vi "BombaPresion.vi"() -> ()   [LabVIEW 2010]
uses:
  <vilib>/Platform/TimedLoop/XDataNode/XDataNode.xnode
  <vilib>/Platform/TimedLoop/XDataNode/timing_clust.ctl
  <vilib>/Platform/TimedLoop/XDataNode/nitl_modes.ctl
  <vilib>/Platform/TimedLoop/XDataNode/wakeup.ctl
  <vilib>/Instr/_visa.llb/VISA Configure Serial Port (Instr).vi
  <vilib>/Platform/TimedLoop/XDataNode/XDNodeRunTimeDep.lvlib
panel:
  out "x*y":dbl
  out "Boolean 2":bool
  out "Boolean":bool
  out "var t 2":i32
  out "nivel presion KPa":dbl(slide) scale=35.0..115.0
  out "presion":dynamicdata(graph)
  in  "presion":dbl(slide) caption="set presion KPa" scale=35.0..115.0
  in  "Period                :":i64=1000
  in  "Flow control    :":u16(ring) items=["None"=0, "XON/XOFF"=1, "RTS/CTS"=2, "DTR/DSR"=4]
  in  "Stop bits         :":u16(ring)=10 items=["1.0"=10, "1.5"=15, "2.0"=20]
  in  "Paridad            :":u16(ring) items=["None", "Odd", "Even", "Mark", "Space"]
  in  "Data bits          :":u16=8 min=5 max=8 step=1
  in  "VISA resource : name:":refnum<visa-resource-name>="COM1"
  in  "Baud rate         :":u32=9600
  in  "stop":bool
  out "Read buffer":string
  # "Sistema Riego"
  # "Configuracion Serial"
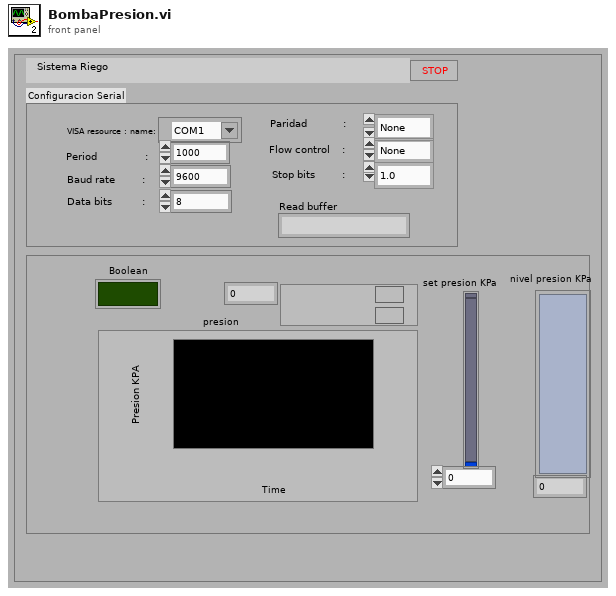
[diagram p1: front panel]
types:
  T1 = typedef "XDNodeRunTimeDep.lvlib/timing_clust.ctl" = cluster{"Expected End [f-1]":u64, "Actual End [f-1]":u64, "Finished Late? [f-1]":bool, "Expected End [i-1]":u64, "Actual End [i-1]":u64, "Finished Late? [i-1]":bool, "Expected Start [i]":u64, "Actual Start [i]":u64, "Expected Start [f]":u64, "Actual Start [f]":u64, "Source Name":string, "Structure Name":string, "Period":i64, "Deadline":i64, "Offset":i64, "Start":i64, "Priority":i32, "Timeout":i32, "Mode":T2, "Wakeup Reason":T3, "Error":errorcluster, "Source Type":string, "Secondary Source Type":string, "Global End Time":u64, "Global Start Time":u64, "Frame Duration":u64, "Iteration Duration":u64, "Assigned CPU":i32, "I/O Scan Engine Mode":u32}
  T2 = typedef "XDNodeRunTimeDep.lvlib/nitl_modes.ctl" = enum32{"No Change", "Process missed periods, maintain original phase", "Discard missed periods, maintain original phase", "Process missed periods, ignore original phase", "Discard missed periods, ignore original phase"}
  T3 = typedef "XDNodeRunTimeDep.lvlib/wakeup.ctl" = enum32{"Normal", "Aborted", "Asynchronous wakeup", "Timing source error", "Timed loop error", "Timeout"}
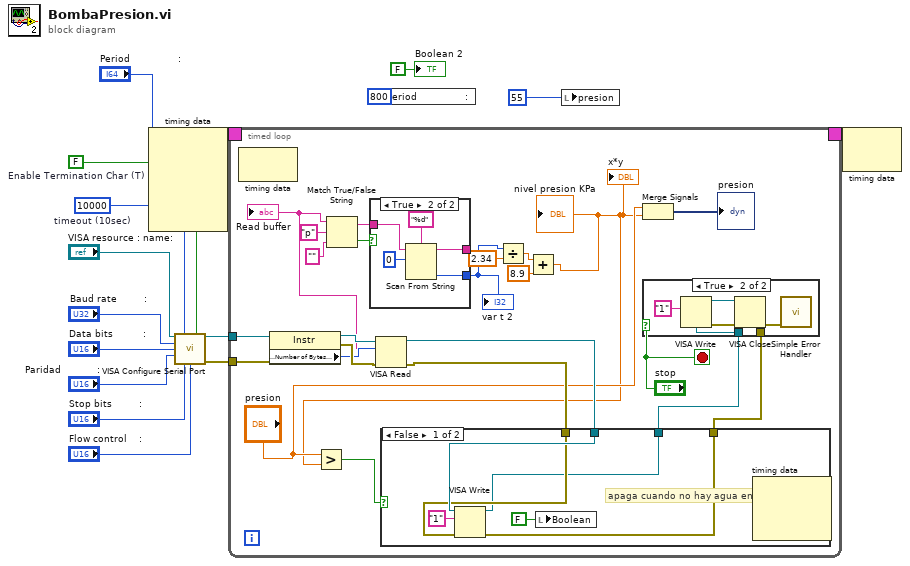
[diagram p0: block diagram]
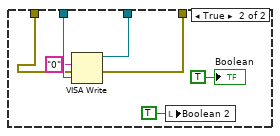
[diagram p2: hidden frame]
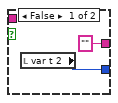
[diagram p3: hidden frame]
diagram:
  w10 = FALSE  # Enable Termination Char (T)
  w11 = u32 10000  # timeout (10sec)
  n1 = node-c288("Period                :") -> (w16:T1)  [unwired: 4 in]
  n2 = call-poly "VISA Configure Serial Port"("VISA resource name"="VISA resource : name:", "timeout (10sec)"=w11, "Enable Termination\nChar (T)"=w10, "baud rate (9600)"="Baud rate         :", "data bits (8)"="Data bits          :", "parity (0:none)"="Paridad            :", "stop bits (10: 1 bit)"="Stop bits         :", "flow control (0:none)"="Flow control    :") -> ("VISA resource name out"=w6:refnum<visa-resource-name>, "error out"=w5:errorcluster)  [unwired: 6 in]
  n3 = timed-loop {
    timing: w16 -> [_]
    timing-out: [_] -> w15
    tunnel: w6 -> [w36]
    tunnel: w5 -> [w35]
    stop <- "stop" stop-if-true
    n4 = node-c288() -> ()  [unwired: 1 in, 1 out]
    n5 = property class="Instr"(reference=w36, error in=w35) -> (reference out=w37:refnum<visa-resource-name>, error out=w39:errorcluster, "Serial Settings:Number of Bytes at Serial Port"=w38:u32)
    n6 = VISA Read(VISA resource name=w37, byte count=w38, error in (no error)=w39) -> (VISA resource name out=w34:refnum<visa-resource-name>, read buffer=w23:string, error out=w33:errorcluster)  [unwired: 1 out]
    "Read buffer" <- w23
    n7 = Match True/False String(2:"" ("false string"), 3:"p" ("true string"), 4:w23) -> (0:w30:bool, 1:w31:string)
    n8 = case shown="True" w30 {
      tunnel: w31 -> [_ w57]
      tunnel: ["" w56] -> _
      tunnel: [w54 w55] -> w20
      frame False {
        n9 = local read "var t 2"() -> (w54:i32)
      }
      frame True {
        n10 = Scan From String(format string="%d", input string=w57, initial scan location=u32 0) -> (remaining string=w56:string, output 1=w55:i32)  [unwired: 2 in, 2 out]
      }
    }
    "var t 2" <- w20
    n11 = Divide(x=w20, y=2.34) -> (x/y=w19:dbl)
    n12 = Add(x=w19, y=8.9) -> (x+y=w17:dbl)
    "nivel presion KPa" <- w17
    "x*y" <- w17
    n13 = Greater?(x="presion", y=w17) -> (0:w22:bool)
    n14 = case shown="False" w22 {
      tunnel: w34 -> [w43 w52]
      tunnel: w33 -> [w42 w51]
      tunnel: [w40 w50] -> w27
      tunnel: [w41 w49] -> w26
      frame False {
        # "apaga cuando no hay agua en pozo"
        n15 = VISA Write(VISA resource name=w43, write buffer="1", error in (no error)=w42) -> (VISA resource name out=w41:refnum<visa-resource-name>, error out=w40:errorcluster)  [unwired: 1 out]
        n16 = local write "Boolean"(FALSE ("Boolean")) -> ()
      }
      frame True {
        n17 = VISA Write(VISA resource name=w52, write buffer="0", error in (no error)=w51) -> (VISA resource name out=w49:refnum<visa-resource-name>, error out=w50:errorcluster)  [unwired: 1 out]
        n18 = local write "Boolean 2"(TRUE ("Boolean 2")) -> ()
        "Boolean" <- TRUE ("Boolean")
      }
    }
    n19 = Merge Signals("presion", w17) -> (→"presion":dynamicdata)
    n20 = case shown="True" "stop" {
      tunnel: w27 -> [_ w62]
      tunnel: w26 -> [_ w61]
      frame False {
      }
      frame True {
        n21 = VISA Write(VISA resource name=w61, write buffer="1", error in (no error)=w62) -> (VISA resource name out=w64:refnum<visa-resource-name>, error out=w63:errorcluster)  [unwired: 1 out]
        n22 = VISA Close(VISA resource name=w64, error in (no error)=w63) -> (error out=w65:errorcluster)
        n23 = call <vilib>:"Simple Error Handler.vi"("error in (no error)"=w65) -> ()  [unwired: 4 in, 5 out]
      }
    }
    n24 = node-c288() -> ()  [unwired: 3 in, 1 out]
  }
  n25 = local write "Period                :"(i64 800 ("Period")) -> ()
  n26 = local write "presion"(u8 55 ("Max Humedad (%)")) -> ()
  n27 = node-c288(w15) -> ()  [unwired: 1 out]
  "Boolean 2" <- FALSE ("Boolean 2")
